vi "get used devices.vi"(8 "error in (no error)":errorcluster caption="Fehler (Eingang, kein Fehler)", 11 "Setup (Eingang)":refnum<class "Setup.lvclass">) -> (0 "error out":errorcluster caption="Fehler (Ausgang)", 2 "used devices":refnum<class "Device.lvclass">[](array[class]), 3 "Setup (Ausgang)":refnum<class "Setup.lvclass">)   [LabVIEW 2013, in "DatenKlassen.lvlib" / "Setup.lvclass"]
uses:
  Setup.lvclass
  Device/Device.lvclass
  Setup.lvclass/Setup.ctl
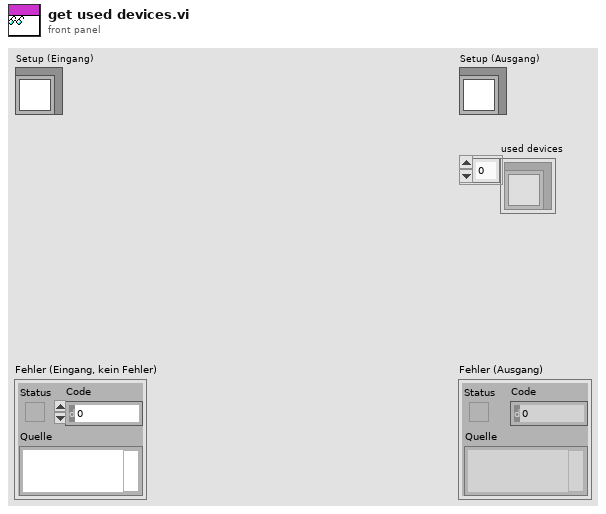
[diagram p1: front panel]
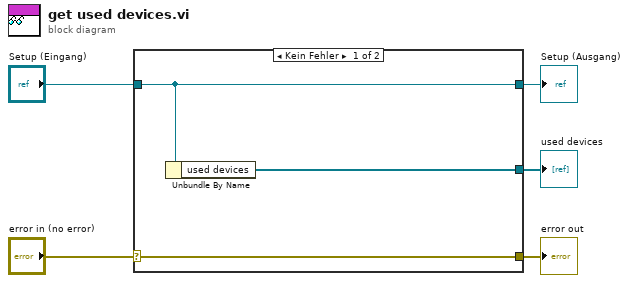
[diagram p0: block diagram]
diagram:
  n1 = case shown="Kein Fehler" "error in (no error)" {
    selector: "error in (no error)" -> [w8 w9]
    tunnel: [w8 w9] -> w4
    tunnel: [w7 w10] -> w2
    tunnel: "Setup (Eingang)" -> [w7 w10]
    tunnel: [w6 _] -> w1
    frame No Error {
      n2 = Unbundle By Name(w7) -> ("used devices"=w6:refnum<class "Device.lvclass">[])
    }
    frame Error {
    }
  }
  "error out" <- w4
  "Setup (Ausgang)" <- w2
  "used devices" <- w1
